vi "ConvertMultiListBoxRefToScheduleArray.vi"(11 "testcaselist ref":refnum<vi>) -> (3 "Array In":string[][](array[string]))   [LabVIEW 2018, in "Library-DataConvert.lvlib"]
uses:
  Library-DataConvert.lvlib
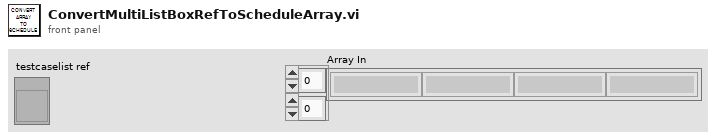
[diagram p1: front panel]
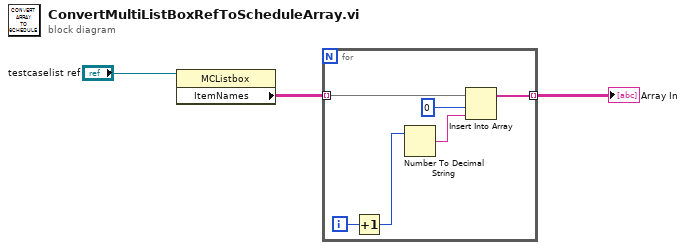
[diagram p0: block diagram]
diagram:
  n1 = property class="MCListbox"(reference="testcaselist ref") -> ("ItemNames"=w2:string[][])  [unwired: 1 in, 2 out]
  n2 = for {
    tunnel: w2 -> [w9] mode=indexing
    tunnel: [w4] -> w1 mode=indexing
    i -> [w8]
    n3 = Increment(x=w8) -> (x+1=w7:i32)
    n4 = Number To Decimal String(number=w7) -> (decimal integer string=w5:string)  [unwired: 1 in]
    n5 = Insert Into Array(array=w9, index=0 ("인덱스"), new element=w5) -> (w4:string[])
  }
  "Array In" <- w1
